vi "GetADSPathsForTwinCAT.vi"() -> ()   [LabVIEW 2022 SP3]
uses:
  <userlib>/Beckhoff-LabVIEW-Interface/_DependsOn/TypeDefs/Low-Levels/Symbol Interface Mode.ctl
panel:
  out "PortInfo":string
  in  "Symbol Interface Mode":T1=enum."Read & Write"
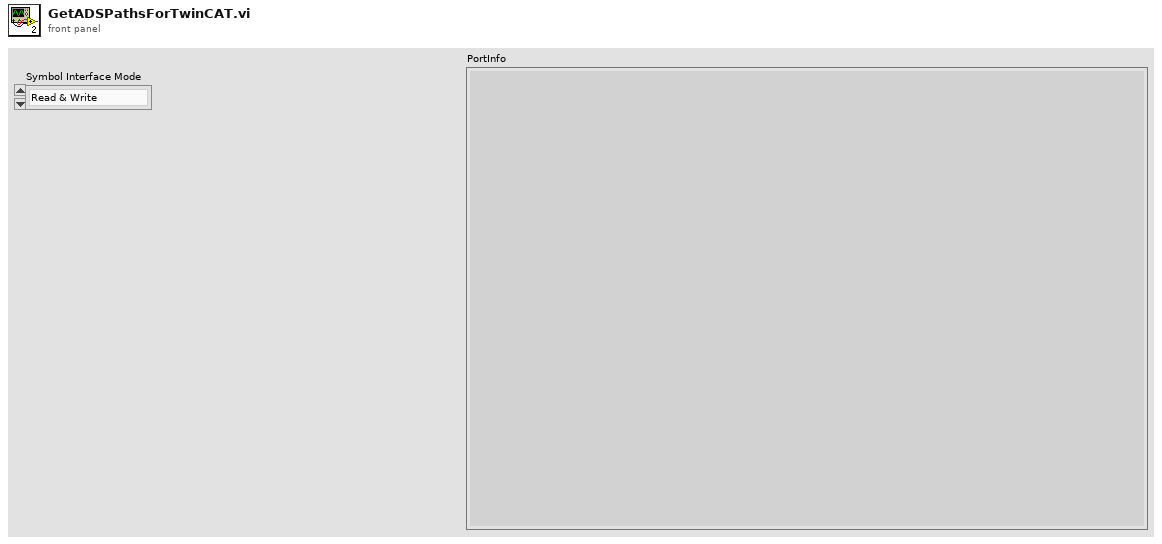
[diagram p1: front panel]
types:
  T1 = typedef "Symbol Interface Mode.ctl" = enum16{"Read Only", "Write Only", "Read & Write"}
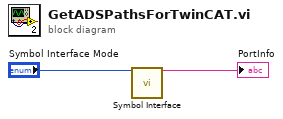
[diagram p0: block diagram]
diagram:
  n1 = call <userlib>:"Symbol Interface.vi"("Symbol Interface Mode"="Symbol Interface Mode") -> ("PortInfo"=→"PortInfo":string)  [unwired: 13 in, 1 out]
